vi "test_readAssembly.vi"() -> ()   [LabVIEW 2023]
uses:
  <vilib>/ethernetip/ethernetip.lvlib
panel:
  out "error out":errorcluster
  out "Data":u8[](array[numeric])=[0, 0, 0, 0, 145, 0, 0, 8, 0, 0, 0, 0, 0, 0, 0, 0, 0, 0, 0, 0, 176, 172, 185, 65, 10, 197, 9, 63, 10, 197, 9, 63, 200, 129, 130, 70, 200, 129, 130, 70, 200, 129, 130, 70]
  in  "Attribute":i32=3 format="%.0x"
  in  "Instance":u32=100 format="%.0x"
  in  "Class":i32=4 format="%.0x"
  in  "Network Path":string="192.168.1.212"
  in  "Timeout (ms)":i32=1000
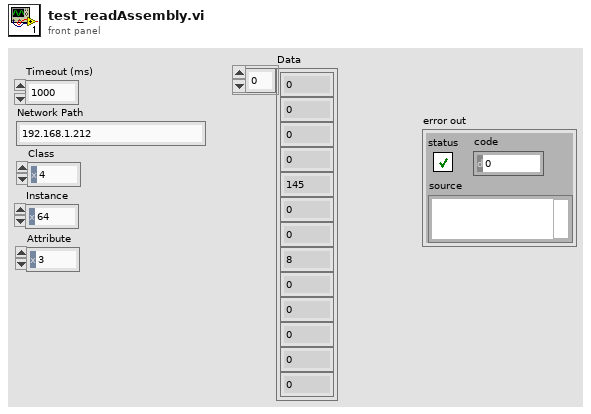
[diagram p1: front panel]
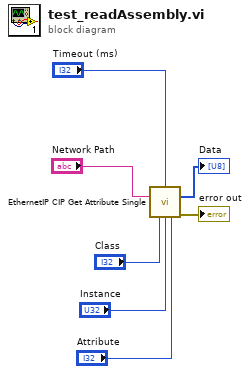
[diagram p0: block diagram]
diagram:
  n1 = call <vilib>:"EthernetIP CIP Get Attribute Single.vi"("Timeout (ms)"="Timeout (ms)", "Network Path"="Network Path", "Class"="Class", "Instance"="Instance", "Attribute"="Attribute") -> ("Data"=→"Data":u8[], "error out"=→"error out":errorcluster)  [unwired: 8 in, 1 out]
